vi "DDVL Find Ctrl Ref.vi"(7 "Control Array":refnum<vi>[](array[refnum]), 13 "Control Label":string="Right Width") -> (8 "Control Ref":refnum<vi>, 15 "Control Found?":bool)   [LabVIEW 2016]
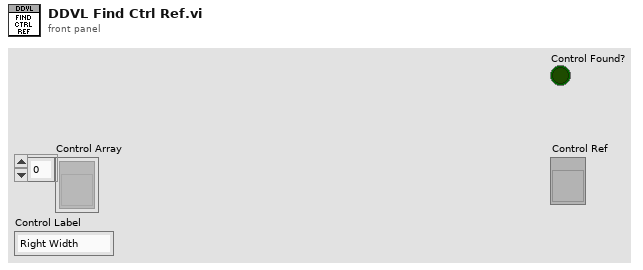
[diagram p1: front panel]
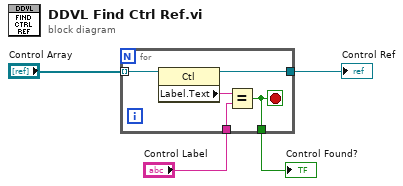
[diagram p0: block diagram]
diagram:
  n1 = for {
    tunnel: "Control Array" -> [w9] mode=indexing
    tunnel: [w7] -> w2
    tunnel: "Control Label" -> [w6]
    tunnel: [w5] -> w1
    stop <- w5 stop-if-true
    n2 = property class="Ctl"(reference=w9) -> (reference out=w7:refnum<vi>, "Label.Text"=w8:string)  [unwired: 1 in, 1 out]
    n3 = Equal?(x=w8, y=w6) -> (x = y?=w5:bool)
  }
  "Control Ref" <- w2
  "Control Found?" <- w1
